vi "AWS-Shared-MD5ofFile.vi"(5 "Local Filepath":path, 7 "Encoding":enum16{"base64", "ASCII Hex"}(ring), 11 "error in":errorcluster) -> (6 "MD5":string, 15 "error out":errorcluster)   [LabVIEW 2012]
uses:
  C:/Users/Jack/repo/aws/AWS-SDK/AWSSDK.dll
  repo/aws/AWS-SDK/AWSSDK.dll
panel:
  # "Inputs"
  # "Outputs"
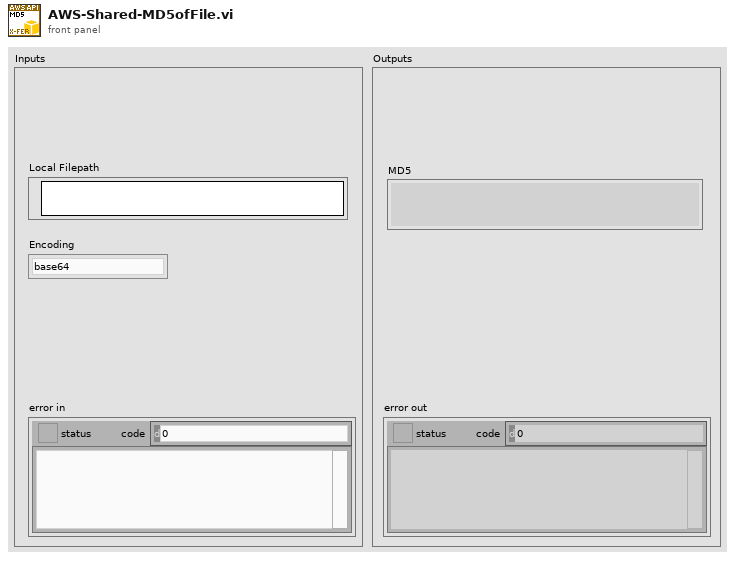
[diagram p1: front panel]
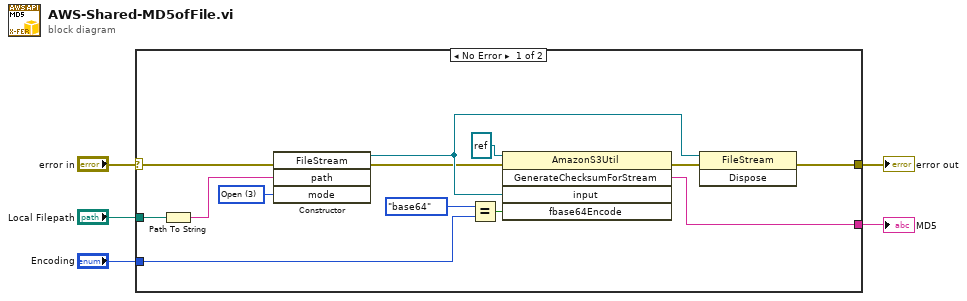
[diagram p0: block diagram]
diagram:
  n1 = case shown="No Error" "error in" {
    selector: "error in" -> [w11 w19]
    tunnel: [w9 w19] -> w5
    tunnel: "Local Filepath" -> [w17 _]
    tunnel: [w15 _] -> w2
    tunnel: "Encoding" -> [w6 _]
    frame No Error {
      w14 = 3 items=["CreateNew"=1, "Create"=2, "Open"=3, "OpenOrCreate"=4, "Truncate"=5, "Append"=6] ("mode")
      n2 = Path To String(path=w17) -> (string=w16:string)
      n3 = constructor class="FileStream"(error in=w11, "path"=w16, "mode"=w14) -> (reference out=w13:refnum<k24>, error out=w10:errorcluster)  [unwired: 2 in, 3 out]
      n4 = Equal?(x=enum16{"base64", "ASCII Hex"}."base64" ("Encoding"), y=w6) -> (x = y?=w7:bool)
      n5 = invoke class="AmazonS3Util" method="GenerateChecksumForStream"(reference=refnum<k24> refnum, error in=w10, "input"=w13, "fbase64Encode"=w7) -> (error out=w12:errorcluster, "GenerateChecksumForStream"=w15:string)  [unwired: 1 in, 3 out]
      n6 = invoke class="FileStream" method="Dispose"(reference=w13, error in=w12) -> (error out=w9:errorcluster)  [unwired: 1 in, 2 out]
    }
    frame Error {
    }
  }
  "error out" <- w5
  "MD5" <- w2
